vi "svx_DAQ_CalculateTiming.vi"(5 "SampClk.MaxRate":dbl=inf, 7 "Display State In":T1={"Channel Info Array"=[], "Timing Mode"=enum."Time", "Timing Control 1"=25600.0, "Timing Control 2"=2560.0, "Timing Control 3"=16, "Timing Indicator 1"=0.1, "Reference Visible?"=FALSE, "Reference Type"=enum."<none>", "Tachometer Channel"="", "Tach Pulses Per Rev"=1, "Tach Direction"=enum."CW", "Tach Slope"=enum."Rising", "Tach Threshold"=0.0, "Trigger Channel"="", "Trigger Level"=20.0, "Pretrigger Samples"=1, "Trigger Slope"=enum."Falling", "Trigger Hysteresis"=0.0, "Logging Visible?"=FALSE, "Enable Logging"=FALSE, "Logfile Path"=path "c:/test.tdms"} caption="State" {"Timing Control 2" format="%#_6f"; "Channel Info Array"."Max" min=0.0 format="± %^#_4g"; "Channel Info Array"."Channel Type" items=["Voltage (V)"=0, "Charge (C)"=9, "-"=99, "SPL (Pa)"=3, "Force (lbf)"=6, "Force (N)"=1, "Acceleration (g) - IEPE"=2, "Acceleration (g) - Charge"=12, "Acceleration (g) - 4 wire DC Voltage"=22, "Velocity (in/s)"=7, "Velocity (mm/s)"=8, "Prox Probe (mil)"=4, "Prox Probe (mm)"=5]}, 11 "error in (no error)":errorcluster) -> (3 "Samples Per Channel":i32, 6 "Sample Rate":dbl, 15 "error out":errorcluster)   [LabVIEW 2017, in "SVX NI-DAQmx AI Configuration XControl.xctl"]
uses:
  <vilib>/addons/Sound and Vibration/svt_DAQmx/Configuration XControl/SVX NI-DAQmx AI Configuration XControl.xctl
  <vilib>/addons/Sound and Vibration/svt_DAQmx/Configuration XControl/SubVIs/svx_DAQ_State.ctl
  <vilib>/addons/Sound and Vibration/svt_DAQmx/Configuration XControl/Controls/svx_DAQ_ChannelInfo.ctl
  <vilib>/addons/Sound and Vibration/svt_DAQmx/Configuration XControl/Controls/svx_DAQ_ChannelType.ctl
  <vilib>/addons/Sound and Vibration/svt_DAQmx/Configuration XControl/Controls/svx_DAQ_Coupling.ctl
  <vilib>/addons/Sound and Vibration/svt_DAQmx/Configuration XControl/Controls/svx_DAQ_Excitation.ctl
  <vilib>/addons/Sound and Vibration/svt_DAQmx/Configuration XControl/Controls/svx_DAQ_TimingType.ctl
  <vilib>/addons/Sound and Vibration/svt_DAQmx/Configuration XControl/Controls/svx_DAQ_ReferenceType.ctl
  <vilib>/addons/Sound and Vibration/svt_DAQmx/Configuration XControl/Controls/svx_DAQ_RotationDirection.ctl
  <vilib>/addons/Sound and Vibration/svt_DAQmx/Configuration XControl/Controls/svx_DAQ_Tach_Slope.ctl
  <vilib>/addons/Sound and Vibration/svt_DAQmx/Configuration XControl/Controls/svx_DAQ_Trigger_Slope.ctl
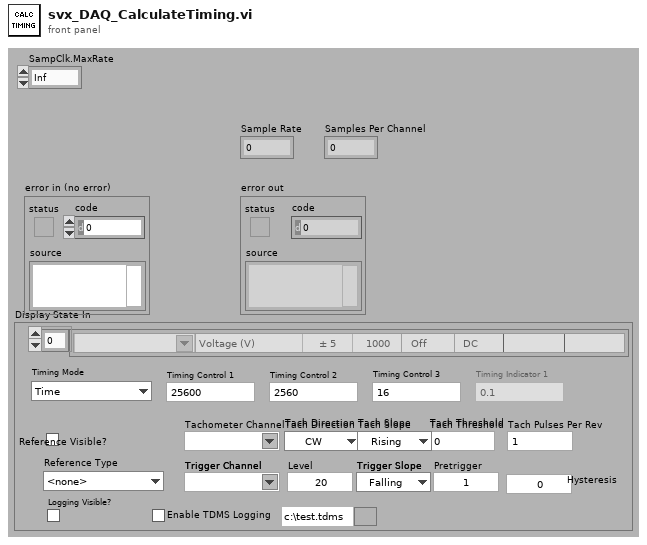
[diagram p1: front panel]
types:
  T1 = typedef "SVX NI-DAQmx AI Configuration XControl.xctl/svx_DAQ_State.ctl" = cluster{"Channel Info Array":T2[], "Timing Mode":T6, "Timing Control 1":dbl, "Timing Control 2":dbl, "Timing Control 3":i32, "Timing Indicator 1":dbl, "Reference Visible?":bool, "Reference Type":T7, "Tachometer Channel":string, "Tach Pulses Per Rev":i32, "Tach Direction":T8, "Tach Slope":T9, "Tach Threshold":dbl, "Trigger Channel":string, "Trigger Level":dbl, "Pretrigger Samples":i32, "Trigger Slope":T10, "Trigger Hysteresis":dbl, "Logging Visible?":bool, "Enable Logging":bool, "Logfile Path":path}
  T2 = typedef "SVX NI-DAQmx AI Configuration XControl.xctl/svx_DAQ_ChannelInfo.ctl" = cluster{"Initialized?":bool, "DAQmx Channel":tag, "Channel Type":T3, "Max":dbl, "Sensitivity":dbl, "Excitation":bool, "Coupling":T4, "Location":string, "Orientation":string, "excitation":T5}
  T3 = typedef "SVX NI-DAQmx AI Configuration XControl.xctl/svx_DAQ_ChannelType.ctl" = u16
  T4 = typedef "SVX NI-DAQmx AI Configuration XControl.xctl/svx_DAQ_Coupling.ctl" = enum16{"AC", "DC"}
  T5 = typedef "svx_DAQ_Excitation.ctl" = enum16{"Off", "Min", "Max"}
  T6 = typedef "SVX NI-DAQmx AI Configuration XControl.xctl/svx_DAQ_TimingType.ctl" = enum16{"Time", "Frequency", "Order"}
  T7 = typedef "SVX NI-DAQmx AI Configuration XControl.xctl/svx_DAQ_ReferenceType.ctl" = enum16{"<none>", "Analog Tachometer", "Analog SW Trigger"}
  T8 = typedef "SVX NI-DAQmx AI Configuration XControl.xctl/svx_DAQ_RotationDirection.ctl" = enum16{"CW", "CCW"}
  T9 = typedef "SVX NI-DAQmx AI Configuration XControl.xctl/svx_DAQ_Tach_Slope.ctl" = enum16{"Rising", "Falling"}
  T10 = typedef "SVX NI-DAQmx AI Configuration XControl.xctl/svx_DAQ_Trigger_Slope.ctl" = enum16{"Falling", "Rising"}
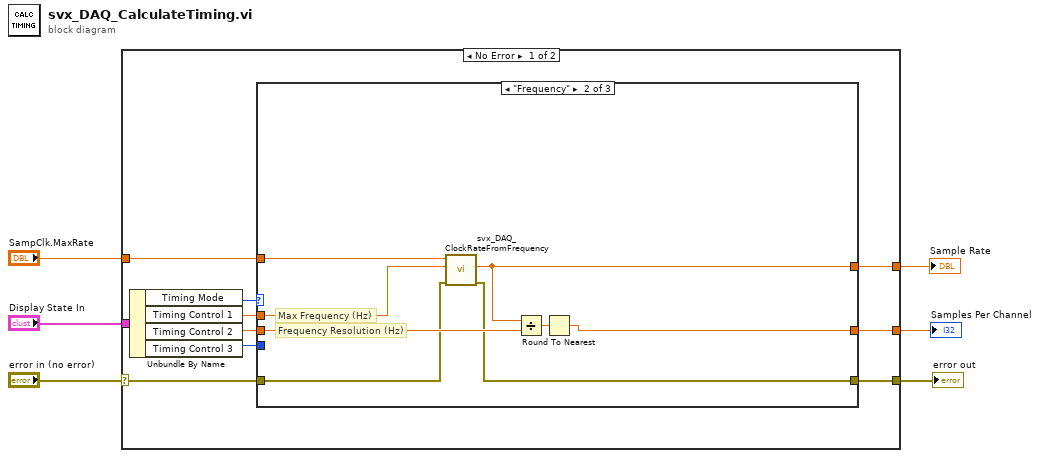
[diagram p0: block diagram]
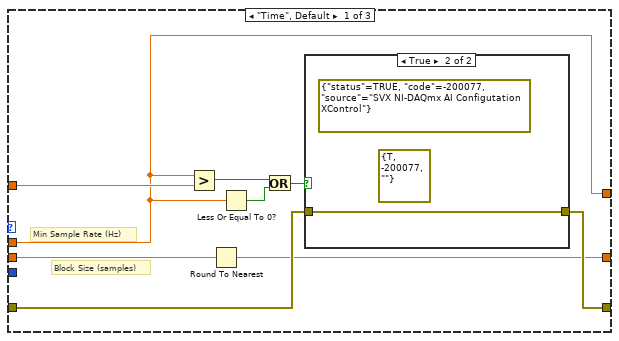
[diagram p2: hidden frame]
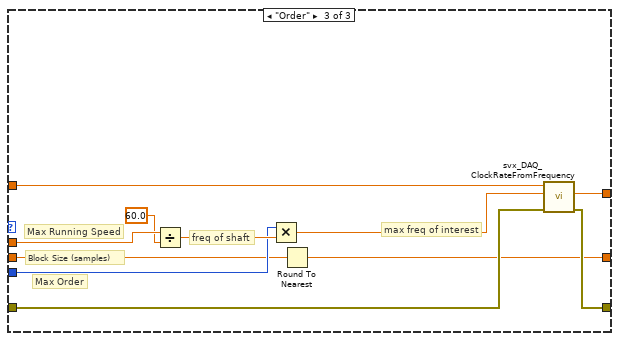
[diagram p4: hidden frame]
diagram:
  n1 = case shown="No Error" "error in (no error)" {
    selector: "error in (no error)" -> [w7 w48]
    tunnel: "Display State In" -> [w16 _]
    tunnel: [w15 w47] -> w5
    tunnel: [w14 w47] -> w4
    tunnel: [w13 w48] -> w3
    tunnel: "SampClk.MaxRate" -> [w12 w47]
    frame No Error {
      n2 = Unbundle By Name(w16) -> ("Timing Mode"=w11:T6, "Timing Control 1"=w10:dbl, "Timing Control 2"=w9:dbl, "Timing Control 3"=w8:i32)
      n3 = case shown="\"Frequency\"" w11 {
        tunnel: w10 -> [w18 w31 w38]
        tunnel: w9 -> [w25 w35 w44]
        tunnel: w8 -> [_ _ w45]
        tunnel: [w18 w30 w41] -> w15
        tunnel: [w17 w33 w36] -> w14
        tunnel: w12 -> [w24 w32 w43]
        tunnel: w7 -> [w20 w29 w40]
        tunnel: [w19 w28 w39] -> w13
        frame "Time", Default {
          # "Block Size (samples)"
          # "Min Sample Rate (Hz)"
          n4 = Greater?(x=w18, y=w24) -> (0:w22:bool)
          n5 = Round To Nearest(number=w25) -> (nearest integer value=w17:dbl)
          n6 = Less Or Equal To 0?(x=w18) -> (x <= 0?=w21:bool)
          n7 = Or(x=w22, y=w21) -> (x .or. y?=w23:bool)
          n8 = case shown="True" w23 {
            tunnel: w20 -> [w26 w27]
            tunnel: [w26 w27] -> w19
            frame False {
            }
            frame True {
              (unwired) errorcluster {"status"=TRUE, "code"=-200077, "source"=""} ("error IO")
              (unwired) errorcluster {"status"=TRUE, "code"=-200077, "source"="SVX NI-DAQmx AI Configutation XControl"} ("error IO")
            }
          }
        }
        frame "Frequency" {
          # "Frequency Resolution (Hz)"
          # "Max Frequency (Hz)"
          n9 = call <vilib>:"svx_DAQ_ClockRateFromFrequency.vi"("error in (no error)"=w29, "Max Frequency of Interest"=w31, "Device Max Sample Rate"=w32) -> ("error out"=w28:errorcluster, "Sample Clock Rate"=w30:dbl)  [unwired: 7 in]
          n10 = Divide(x=w30, y=w35) -> (x/y=w34:dbl)
          n11 = Round To Nearest(number=w34) -> (nearest integer value=w33:dbl)
        }
        frame "Order" {
          # "Max Order"
          # "Block Size (samples)"
          # "Max Running Speed"
          # "max freq of interest"
          # "freq of shaft"
          n12 = Divide(x=w38, y=60.0 ("x")) -> (x/y=w46:dbl)
          n13 = Multiply(x=w45, y=w46) -> (x*y=w42:dbl)
          n14 = Round To Nearest(number=w44) -> (nearest integer value=w36:dbl)
          n15 = call <vilib>:"svx_DAQ_ClockRateFromFrequency.vi"("error in (no error)"=w40, "Max Frequency of Interest"=w42, "Device Max Sample Rate"=w43) -> ("error out"=w39:errorcluster, "Sample Clock Rate"=w41:dbl)  [unwired: 7 in]
        }
      }
    }
    frame Error {
    }
  }
  "Samples Per Channel" <- w4
  "Sample Rate" <- w5
  "error out" <- w3
